vi "Write ClockT0.vi"(8 "error in (no error)":errorcluster, 10 "ClockT0":u64, 11 "CIFCorePlugin in":refnum<class "CIFCorePlugin.lvclass">) -> (0 "error out":errorcluster, 3 "CIFCorePlugin out":refnum<class "CIFCorePlugin.lvclass">)   [LabVIEW 2021, in "CIFCorePlugin.lvclass"]
doc: "Update the timestamp. Time is U64, absolute time in nS in the appropriate clockID configured for the plugin."
uses:
  CIFCorePlugin.lvclass
  CIFCorePlugin.lvclass/CIFCorePlugin.ctl
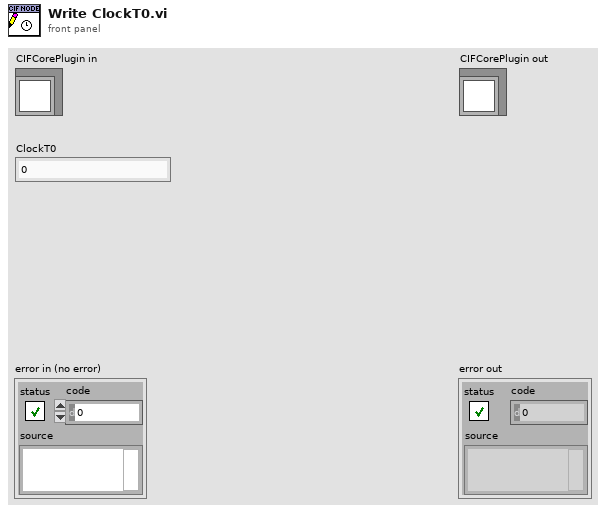
[diagram p1: front panel]
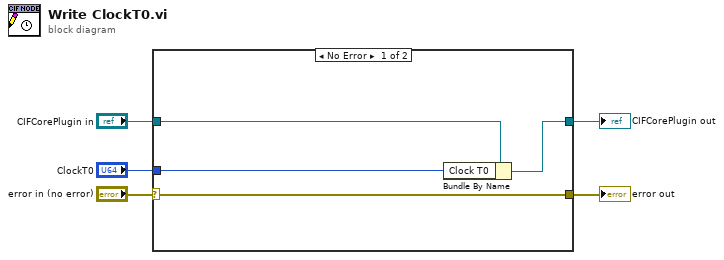
[diagram p0: block diagram]
diagram:
  n1 = case shown="No Error" "error in (no error)" {
    selector: "error in (no error)" -> [w6 w10]
    tunnel: [w6 w10] -> w4
    tunnel: [w9 w11] -> w2
    tunnel: "CIFCorePlugin in" -> [w8 w11]
    tunnel: "ClockT0" -> [w7 _]
    frame No Error {
      n2 = Bundle By Name(cluster=w8, "Clock T0"=w7) -> (w9:refnum<class "CIFCorePlugin.lvclass">)
    }
    frame Error {
    }
  }
  "error out" <- w4
  "CIFCorePlugin out" <- w2
